vi "Increment Assert Count.vi"(8 "error in (no error)":errorcluster, 11 "Standard Display Configuration in":refnum<class "Standard Display Configuration.lvclass">) -> (0 "error out":errorcluster, 2 "Assert Count Value":i32, 3 "Standard Display Configuration out":refnum<class "Standard Display Configuration.lvclass">)   [LabVIEW 2018, in "Assert API Components.lvlib" / "Assert Display.lvlib" / "Main Display.lvlib" / "Standard Display Configuration.lvclass"]
doc: "Increments the Assert Count and writes it to the private data of the class - also outputs the count value for further use."
uses:
  Standard Display Configuration.lvclass
  C:/Users/UKHornP/Documents/Work/Projects/Assert API/Core/Main Display/Display Configurations/Base Display Configuration.lvclass
  Base Display Configuration.lvclass/Base Display Configuration.ctl
  Base Display Configuration.lvclass
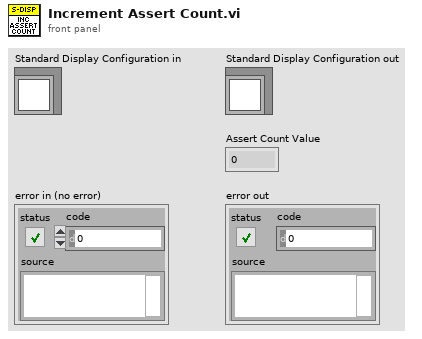
[diagram p1: front panel]
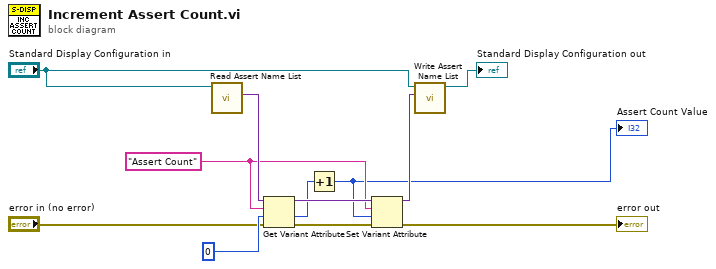
[diagram p0: block diagram]
diagram:
  w4 = "Assert Count" ("name")
  n1 = call "Read Assert Name List.vi"("Base Display Configuration in"="Standard Display Configuration in") -> ("Assert Name List"=w8:variant)  [unwired: 10 in]
  n2 = Get Variant Attribute(Variant=w8, name=w4, default value (empty Variant)=0, error in="error in (no error)") -> (duplicate Variant=w9:variant, value=w6:i32, error out=w12:errorcluster)  [unwired: 1 out]
  n3 = Increment(x=w6) -> (x+1=w1:i32)
  "Assert Count Value" <- w1
  n4 = Set Variant Attribute(Variant=w9, name=w4, value=w1, error in=w12) -> (Variant out=w11:variant, error out=→"error out":errorcluster)  [unwired: 1 out]
  n5 = call "Write Assert Name List.vi"("Assert Name List"=w11, "Base Display Configuration in"="Standard Display Configuration in") -> ("Base Display Configuration out"=→"Standard Display Configuration out":refnum<class "Standard Display Configuration.lvclass">)  [unwired: 9 in]
